vi "string to msgpack.vi"(11 "String":string) -> (3 "msgpack":u8[](array[numeric]) format="%x")   [LabVIEW 2020, in "wamplv.lvlib" / "MessagePack.lvclass"]
uses:
  MessagePack.lvclass
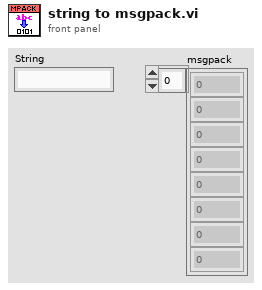
[diagram p1: front panel]
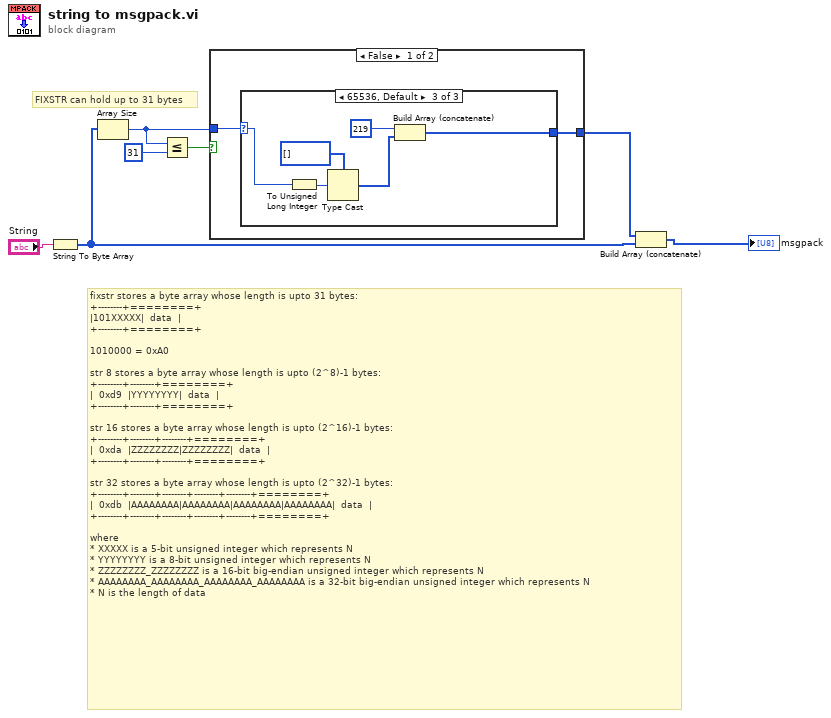
[diagram p0: block diagram]
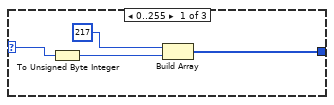
[diagram p2: hidden frame]
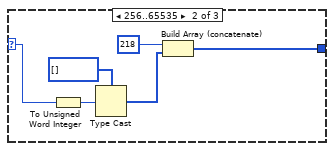
[diagram p3: hidden frame]
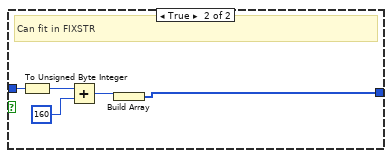
[diagram p4: hidden frame]
diagram:
  # "fixstr stores a byte array whose length is upto 31 bytes:\n+--------+========+\n|101XXXXX|  data  |\n+--------+========+\n\n1010000 = 0xA0\n\nstr 8 stores a byte array whose length is upto (2^8)-1 bytes:\n+--------+--------+========+\n|  0xd9  |YYYYYYYY|  data  |\n+--------+--------+========+\n\nstr 16 stores a byte array whose length is upto (2^16)-1 bytes:\n+--------+--------+--------+========+\n|  0xda  |ZZZZZZZZ|ZZZZZZZZ|  data  |\n+--------+--------+--------+========+\n\nstr 32 stores a byte array whose length is upto (2^32)-1 bytes:\n+--------+--------+--------+--------+--------+========+\n|  0xdb  |AAAAAAAA|AAAAAAAA|AAAAAAAA|AAAAAAAA|  data  |\n+--------+--------+--------+--------+--------+========+\n\nwhere\n* XXXXX is a 5-bit unsigned integer which represents N\n* YYYYYYYY is a 8-bit unsigned integer which represents N\n* ZZZZZZZZ_ZZZZZZZZ is a 16-bit big-endian unsigned integer which represents N\n* AAAAAAAA_AAAAAAAA_AAAAAAAA_AAAAAAAA is a 32-bit big-endian unsigned integer which represents N\n* N is the length of data"
  # "FIXSTR can hold up to 31 bytes"
  n1 = String To Byte Array(string="String") -> (unsigned byte array=w4:u8[])
  n2 = Array Size(array=w4) -> (size(s)=w3:i32)
  n3 = Less Or Equal?(x=w3, y=31) -> (x <= y?=w5:bool)
  n4 = case shown="False" w5 {
    tunnel: w3 -> [w9 w30]
    tunnel: [w8 w26] -> w2
    frame False {
      n5 = case shown="65536, Default" w9 {
        selector: w9 -> [w13 w17 w20]
        tunnel: [w10 w18 w24] -> w8
        frame 0..255 {
          n6 = To Unsigned Byte Integer(number=w13) -> (unsigned 8bit integer=w11:u8)
          n7 = Build Array(u8 217 ("y"), w11) -> (w10:u8[])
        }
        frame 256..65535 {
          n8 = To Unsigned Word Integer(number=w17) -> (unsigned 16bit integer=w15:u16)
          n9 = Type Cast(type=u8[] [] ("bytes"), x=w15) -> (*(type *) &x=w14:u8[])
          n10 = Build Array (concatenate)(u8 218 ("y"), w14) -> (w18:u8[])
        }
        frame 65536, Default {
          n11 = To Unsigned Long Integer(number=w20) -> (unsigned 32bit integer=w21:u32)
          n12 = Type Cast(type=u8[] [] ("bytes"), x=w21) -> (*(type *) &x=w22:u8[])
          n13 = Build Array (concatenate)(u8 219 ("y"), w22) -> (w24:u8[])
        }
      }
    }
    frame True {
      # "Can fit in FIXSTR"
      n14 = To Unsigned Byte Integer(number=w30) -> (unsigned 8bit integer=w29:u8)
      n15 = Add(x=w29, y=u8 160) -> (x+y=w27:u8)
      n16 = Build Array(w27) -> (w26:u8[])
    }
  }
  n17 = Build Array (concatenate)(w2, w4) -> (→"msgpack":u8[])
